vi "SetProgress.vi"(8 "error in (no error)":errorcluster, 9 "SubStep":dbl, 10 "ProgressBarCluster":T1) -> (0 "error out":errorcluster)   [LabVIEW 2014, in "CS++MessagemakerUtilities.lvlib"]
uses:
  CS++MessagemakerUtilities.lvlib
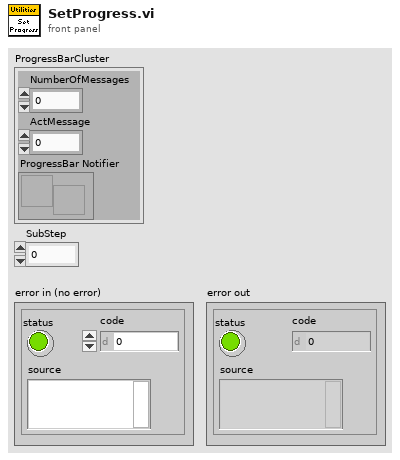
[diagram p1: front panel]
types:
  T1 = cluster{"NumberOfMessages":u16, "ActMessage":u16, "ProgressBar Notifier":refnum<notifier>}
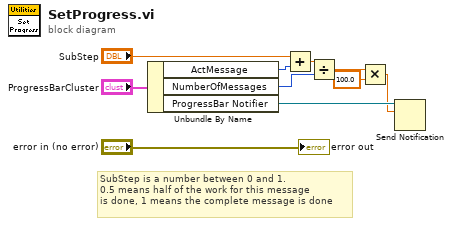
[diagram p0: block diagram]
diagram:
  # "SubStep is a number between 0 and 1.\n0.5 means half of the work for this message\nis done, 1 means the complete message is done"
  n1 = Unbundle By Name("ProgressBarCluster") -> ("ActMessage"=w6:u16, "NumberOfMessages"=w8:u16, "ProgressBar Notifier"=w9:refnum<notifier>)
  n2 = Add(x="SubStep", y=w6) -> (x+y=w7:dbl)
  n3 = Divide(x=w7, y=w8) -> (x/y=w3:dbl)
  n4 = Multiply(x=w3, y=100.0) -> (x*y=w2:dbl)
  n5 = Send Notification(notification=w2, notifier=w9) -> ()  [unwired: 1 in, 2 out]
  "error out" <- "error in (no error)"
